vi "iWorx Get Visible Chart Array Data.vi"(7 "Waveform Chart 3":refnum<vi>, 8 "Error In":errorcluster) -> (0 "Error Out":errorcluster, 2 "Waveforms Out":waveform(dbl)[](array[waveform]))   [LabVIEW 2012]
uses:
  <vilib>/Waveform/WDTOps.llb/WDT Get Waveform Subset DBL.vi
  <vilib>/Waveform/WDTOps.llb/WDT Append Waveforms DBL.vi
panel:
  out "size(s) 2":i32
  out "size(s)":i32[](array[numeric])
  out "Lengths":i32[](array[numeric])
  out "t0":timestamp
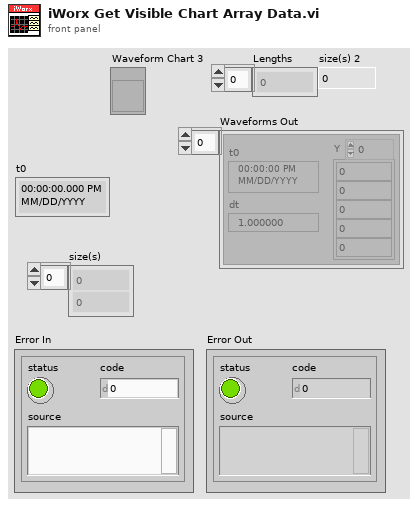
[diagram p1: front panel]
types:
  T1 = typedef "LVRangeTypeDef.ctl" = cluster{"Minimum":dbl, "Maximum":dbl, "Increment":dbl, "Minor Increment":dbl, "Start":dbl}
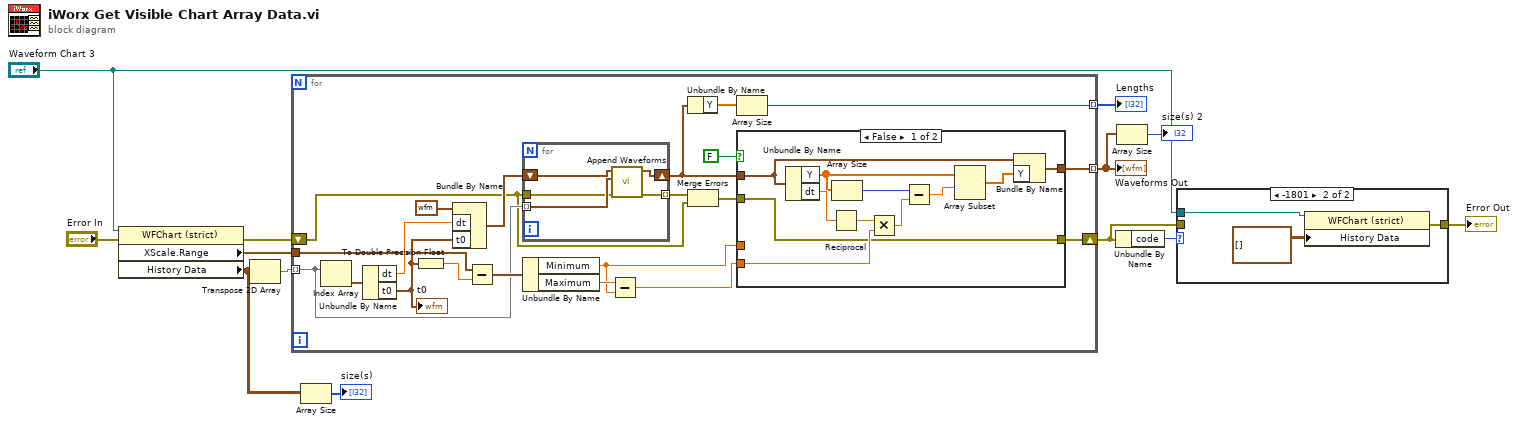
[diagram p0: block diagram]
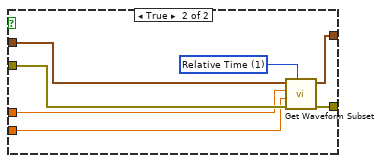
[diagram p2: hidden frame]
diagram:
  n1 = property class="WFChart (strict)"(reference="Waveform Chart 3", error in="Error In") -> (error out=w10:errorcluster, "XScale.Range"=w11:T1, "History Data"=w4:waveform(dbl)[][])  [unwired: 1 out]
  n2 = Transpose 2D Array(2D array=w4) -> (transposed array=w3:waveform(dbl)[][])
  n3 = for {
    tunnel: w3 -> [w23] mode=indexing
    tunnel: w11 -> [w19]
    tunnel: [w15] -> w2 mode=indexing
    shift-right: [w25] -> w12
    shift-left: w10 -> [w16]
    tunnel: [w14] -> w6 mode=indexing
    n4 = Index Array(array=w23) -> (element=w22:waveform(dbl))  [unwired: 1 in]
    n5 = Unbundle By Name(w22) -> ("dt"=w29:dbl, "t0"=w28:timestamp)
    "t0" <- w28
    n6 = To Double Precision Float(number=w28) -> (double precision float=w26:dbl)
    n7 = Bundle By Name(cluster=waveform(dbl) {"t0"=timestamp(0 s since 1904-01-01), "dt"=2.267573696145e-05, "Y"=[]} ("waveform out"), "dt"=w29, "t0"=w28) -> (w31:waveform(dbl))
    n8 = Subtract(x=w19, y=w26) -> (x-y=w27:T1)
    n9 = for {
      tunnel: w23 -> [w56] mode=indexing
      shift-right: [w57] -> w21
      shift-left: w31 -> [w55]
      tunnel: w16 -> [w54]
      tunnel: [w53] -> w32 mode=indexing
      n10 = call-poly <vilib>:"Append Waveforms.vi"("error in (no error)"=w54, "waveform B"=w56, "waveform A"=w55) -> ("error out"=w53:errorcluster, "waveform out"=w57:waveform(dbl))  [unwired: 7 in]
    }
    n11 = Unbundle By Name(w27) -> ("Minimum"=w20:dbl, "Maximum"=w30:dbl)
    n12 = Subtract(x=w30, y=w20) -> (x-y=w18:dbl)
    n13 = Unbundle By Name(w21) -> ("Y"=w24:dbl[])
    n14 = Merge Errors(w32, w16) -> (w33:errorcluster)
    n15 = Array Size(array=w24) -> (size(s)=w14:i32)
    n16 = case shown="False" FALSE {
      tunnel: w33 -> [w35 w52]
      tunnel: [w35 w50] -> w25
      tunnel: [w36 w49] -> w15
      tunnel: w21 -> [w39 w48]
      tunnel: w20 -> [_ w47]
      tunnel: w18 -> [w44 w46]
      frame False {
        n17 = Unbundle By Name(w39) -> ("Y"=w40:dbl[], "dt"=w42:dbl)
        n18 = Reciprocal(x=w42) -> (1/x=w41:dbl)
        n19 = Array Size(array=w40) -> (size(s)=w45:i32)
        n20 = Multiply(x=w41, y=w44) -> (x*y=w43:dbl)
        n21 = Subtract(x=w45, y=w43) -> (x-y=w37:dbl)
        n22 = Array Subset(array=w40, index=w37) -> (w38:dbl[])  [unwired: 1 in]
        n23 = Bundle By Name(cluster=w39, "Y"=w38) -> (w36:waveform(dbl))
      }
      frame True {
        w51 = u16 1 items=["Samples", "Relative Time"] ("start/duration format")
        n24 = call-poly <vilib>:"Get Waveform Subset.vi"("start/duration format"=w51, "error in (no error)"=w52, "duration"=w46, "start samples/time"=w47, "waveform in"=w48) -> ("error out"=w50:errorcluster, "waveform out"=w49:waveform(dbl))  [unwired: 1 in, 2 out]
      }
    }
  }
  "Lengths" <- w6
  "Waveforms Out" <- w2
  n25 = Array Size(array=w4) -> (size(s)=→"size(s)":i32[])
  n26 = Unbundle By Name(w12) -> ("code"=w13:i32)
  n27 = Array Size(array=w2) -> (size(s)=→"size(s) 2":i32)
  n28 = case shown="-1801" w13 {
    tunnel: "Waveform Chart 3" -> [_ w61]
    tunnel: w12 -> [w58 _]
    tunnel: [w58 w60] -> w8
    frame 0, Default {
    }
    frame -1801 {
      n29 = property class="WFChart (strict)"(reference=w61, "History Data"=waveform(dbl)[][] []) -> (error out=w60:errorcluster)  [unwired: 1 in, 1 out]
    }
  }
  "Error Out" <- w8
